vi "PathToRezult.vi"() -> (3 "pathToRezult":path)   [LabVIEW 2017]
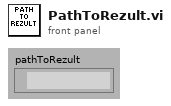
[diagram p1: front panel]
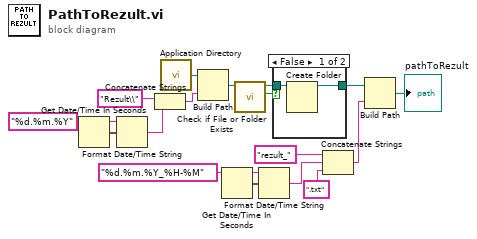
[diagram p0: block diagram]
diagram:
  n1 = Get Date/Time In Seconds() -> (seconds since 1Jan1904=w10:timestamp)
  n2 = Format Date/Time String(time format string (%c)="%d.%m.%Y", seconds (now)=w10) -> (date/time string=w11:string)  [unwired: 1 in]
  n3 = Concatenate Strings("Rezult\\" ("prompt (Create Folder)"), w11) -> (w8:string)
  n4 = call <vilib>:"Application Directory.vi"() -> ("Application Directory"=w2:path)
  n5 = Build Path(base path=w2, name or relative path=w8) -> (appended path=w3:path)
  n6 = Get Date/Time In Seconds() -> (seconds since 1Jan1904=w14:timestamp)
  n7 = call <vilib>:"Check if File or Folder Exists.vi"("path"=w3) -> ("file or folder exists?"=w4:bool, "dup path"=w5:path)  [unwired: 8 in, 1 out]
  n8 = Format Date/Time String(time format string (%c)="%d.%m.%Y_%H-%M", seconds (now)=w14) -> (date/time string=w15:string)  [unwired: 1 in]
  n9 = case shown="False" w4 {
    tunnel: w5 -> [w19 w20]
    tunnel: [w18 w20] -> w6
    frame False {
      n10 = Create Folder(path (use dialog)=w19) -> (created path=w18:path)  [unwired: 2 in, 2 out]
    }
    frame True {
    }
  }
  n11 = Concatenate Strings("rezult_" ("name or relative path"), w15, ".txt" ("string")) -> (w17:string)
  n12 = Build Path(base path=w6, name or relative path=w17) -> (appended path=→"pathToRezult":path)
